vi "fgv_linear_vel_buffer.vi"(7 "agv_cmd_angle":enum16{"ini", "write", "read"}(ring), 9 "index":i32, 10 "linear_vel in":dbl, 11 "dim size":i32) -> (3 "linear_vel out":dbl)   [LabVIEW 2019]
uses:
  <vilib>/Analysis/baseanly.llb/Mean (DBL).vi
  <vilib>/Analysis/NI_AALBase.lvlib
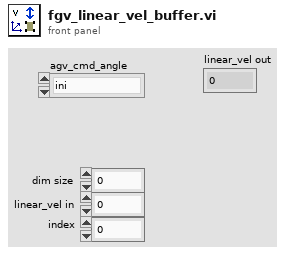
[diagram p1: front panel]
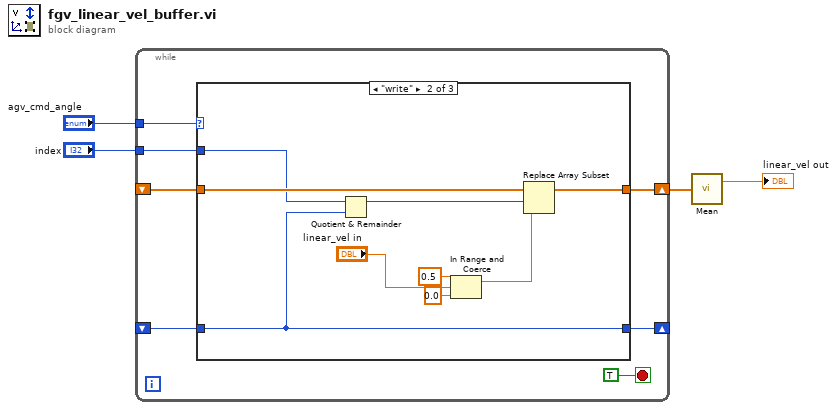
[diagram p0: block diagram]
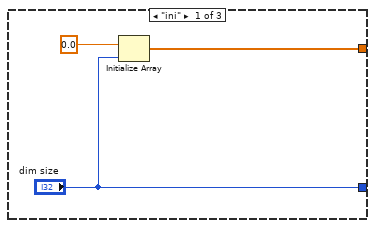
[diagram p2: hidden frame]
diagram:
  n1 = while {
    tunnel: "agv_cmd_angle" -> [w10]
    shift-right: [w9] -> w3
    shift-left: _ -> [w8]
    tunnel: "index" -> [w7]
    shift-right: [w6] -> _
    shift-left: _ -> [w5]
    stop <- TRUE stop-if-true
    n2 = case shown="\"write\"" w10 {
      tunnel: [w13 w22 w25] -> w9
      tunnel: w8 -> [_ w23 w25]
      tunnel: w7 -> [_ w20 _]
      tunnel: ["dim size" w19 w24] -> w6
      tunnel: w5 -> [_ w19 w24]
      frame "ini" {
        n3 = Initialize Array(0.0 ("원소"), "dim size") -> (w13:dbl[])
      }
      frame "write" {
        n4 = Quotient & Remainder(x=w20, y=w19) -> (x-y*floor(x/y)=w21:i32)  [unwired: 1 out]
        n5 = In Range and Coerce(upper limit=0.5 ("상위 리미트"), x="linear_vel in", lower limit=0.0 ("하위 리미트")) -> (coerced(x)=w17:dbl)  [unwired: 1 out]
        n6 = Replace Array Subset(array=w23, new element=w17, index=w21) -> (w22:dbl[])
      }
      frame "read", Default {
      }
    }
  }
  n7 = call-poly <vilib>:"Mean.vi"("X"=w3) -> ("mean"=→"linear_vel out":dbl)  [unwired: 1 out]
